vi "649Set.vi"() -> ()   [LabVIEW 2022 SP3]
uses:
  <vilib>/numeric/Random Number (Range) U64.vi
  <vilib>/numeric/sub_Random U32.vi
  <vilib>/Utility/file.llb/Write Delimited Spreadsheet (string).vi
panel:
  in  "append to file?":bool
  in  "?":bool
  in  "file path (dialog if empty)":path
  out "?":string[][](array[string])
  # "6@49"
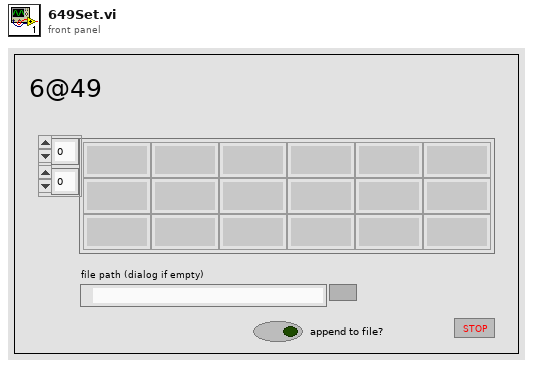
[diagram p1: front panel]
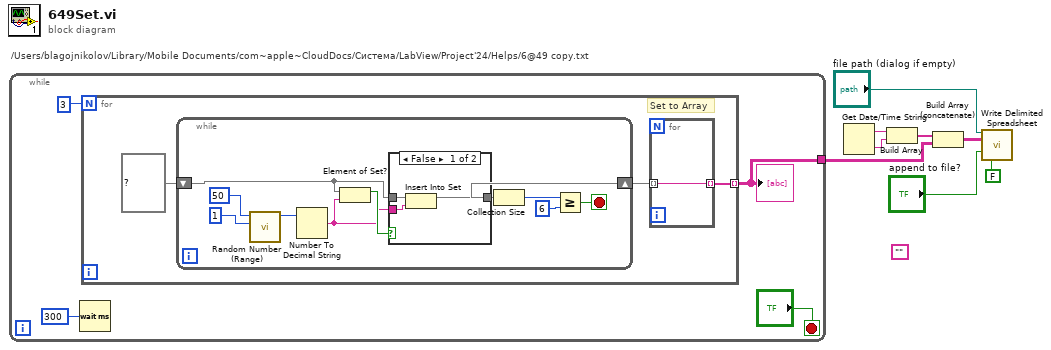
[diagram p0: block diagram]
diagram:
  (unwired) ""
  # "/Users/blagojnikolov/Library/Mobile Documents/com~apple~CloudDocs/Система/LabView/Project'24/Helps/6@49 copy.txt"
  n1 = while {
    tunnel: [w11] -> w8
    stop <- "?" stop-if-true
    n2 = Wait (ms)(milliseconds to wait=u32 300) -> ()  [unwired: 1 out]
    n3 = for {
      N: 3 -> [_]
      tunnel: [w13] -> w11 mode=indexing
      # "Set to Array"
      n4 = while {
        shift-right: [w20] -> w14
        shift-left: set{string} {} ("Set") -> [w22]
        stop <- w17 stop-if-true
        n5 = call-poly <vilib>:"Random Number (Range).vi"("lower bound (0)"=u64 1, "upper bound (100)"=u64 50) -> ("number"=w24:u64)  [unwired: 9 in]
        n6 = Number To Decimal String(number=w24) -> (decimal integer string=w21:string)  [unwired: 1 in]
        n7 = Element of Set?(10:w21, 11:w22) -> (3:w23:bool)
        n8 = case shown="False" w23 {
          tunnel: w22 -> [w28 w30]
          tunnel: [w27 w30] -> w20
          tunnel: w21 -> [w29 _]
          frame False {
            n9 = Insert Into Set(10:w29, 11:w28) -> (3:w27:set{string})  [unwired: 1 out]
          }
          frame True {
          }
        }
        n10 = Collection Size(1:w20) -> (0:w19:i32)
        n11 = Greater Or Equal?(x=w19, y=6) -> (x >= y?=w17:bool)
      }
      n12 = for {
        tunnel: [w16] -> w13 mode=indexing
        tunnel: w14 -> [w16] mode=indexing
      }
    }
    "?" <- w11
  }
  n13 = Get Date/Time String() -> (date string=w7:string, time string=w6:string)  [unwired: 3 in]
  n14 = Build Array(w7, w6) -> (w5:string[])
  n15 = Build Array (concatenate)(w5, w8) -> (w4:string[][])
  n16 = call-poly <vilib>:"Write Delimited Spreadsheet.vi"("file path (dialog if empty)"="file path (dialog if empty)", "2D data"=w4, "append to file? (new file:F)"="append to file?", "transpose? (no:F)"=FALSE) -> ()  [unwired: 10 in, 2 out]
